vi "Write Pages Properties.vi"(8 "Error In":errorcluster, 10 "All Pages Properties":T10(array[cluster]), 11 "Custom Device .NET Ref In":refnum<k24>) -> (0 "Error Out":errorcluster, 3 "Custom Device .NET Ref Out":refnum<k24>)   [LabVIEW 2015, in "VeriStand Custom Device XML Parser.lvlib"]
doc: "Write the properties for all items of a page then writes the array of pages to the custom device"
uses:
  VeriStand Custom Device XML Parser.lvlib
  NationalInstruments.VeriStand.XMLReader
  XML Controls/Page Properties.ctl
  XML Controls/Path Cluster.ctl
  XML Controls/Help File Properties.ctl
  XML Controls/ActionVIs Properties.ctl
  XML Controls/ButtonLists Properties.ctl
  XML Controls/Button Type.ctl
  XML Controls/Dependency Properties.ctl
  XML Controls/RunTimeMenus Properties.ctl
  XML Controls/Execution Types.ctl
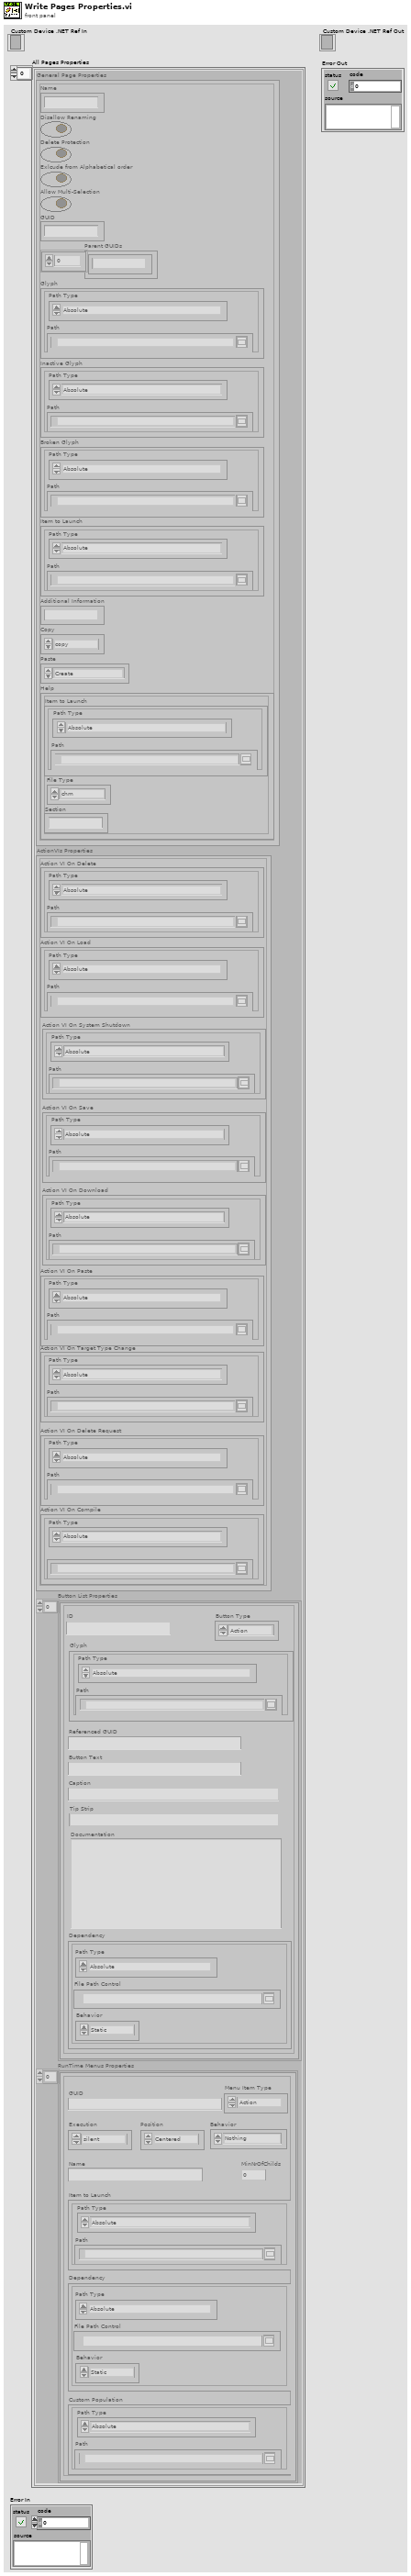
[diagram p1: front panel]
types:
  T1 = typedef "VeriStand Custom Device XML Parser.lvlib/Page Properties.ctl" = cluster{"Name":string, "Disallow Renaming":bool, "Delete Protection":bool, "Exlcude from Alphabetical order":bool, "Allow Multi-Selection":bool, "GUID":string, "Parent GUIDs":string[], "Glyph":T2, "Inactive Glyph":T2, "Broken Glyph":T2, "Item to Launch":T2, "Additional Information":string, "Copy":enum16{"copy", "disabled"}, "Paste":enum16{"Create", "CreatIfNotExists_GUID", "CreatIfNotExists_Name", "Replace", "Dialog"}, "Help":T3}
  T2 = typedef "VeriStand Custom Device XML Parser.lvlib/Path Cluster.ctl" = cluster{"Path":path, "Path Type":enum16{"Absolute", "To Base", "To Common Doc Dir", "To Application Data Dir"}}
  T3 = typedef "VeriStand Custom Device XML Parser.lvlib/Help File Properties.ctl" = cluster{"Item to Launch":T2, "Section":string, "File Type":enum16{"chm", "other"}}
  T4 = typedef "VeriStand Custom Device XML Parser.lvlib/ActionVIs Properties.ctl" = cluster{"Action VI On Delete":T2, "Action VI On Load":T2, "Action VI On Paste":T2, "Action VI On Target Type Change":T2, "Action VI On Delete Request":T2, "Action VI On Compile":T2, "Action VI On System Shutdown":T2, "Action VI On Save":T2, "Action VI On Download":T2}
  T5 = typedef "VeriStand Custom Device XML Parser.lvlib/ButtonLists Properties.ctl" = cluster{"ID":string, "Glyph":T2, "Button Type":T6, "Referenced GUID":string, "Button Text":string, "Caption":string, "Tip Strip":string, "Documentation":string, "Dependency":T7}
  T6 = typedef "VeriStand Custom Device XML Parser.lvlib/Button Type.ctl" = enum16{"Action", "Dialog", "Page", "Notification", "Separator"}
  T7 = typedef "VeriStand Custom Device XML Parser.lvlib/Dependency Properties.ctl" = cluster{"File Path Control":path, "Path Type":enum16{"Absolute", "To Base", "To Common Doc Dir", "To Application Data Dir"}, "Behavior":enum16{"Static", "Dynamic"}}
  T8 = typedef "VeriStand Custom Device XML Parser.lvlib/RunTimeMenus Properties.ctl" = cluster{"GUID":string, "Execution":T9, "MinNrOfChilds":u32, "Name":string, "Item to Launch":T2, "Dependency":T7, "Custom Population":T2, "Menu Item Type":enum16{"Action", "VI", "Separator", "Custom"}, "Behavior":enum16{"Nothing", "Open Front Panel"}, "Position":enum16{"Centered", "Mouse Pointer"}}
  T9 = typedef "VeriStand Custom Device XML Parser.lvlib/Execution Types.ctl" = enum16{"silent", "modal", "floating", "default"}
  T10 = cluster{"General Page Properties":T1, "ActionVIs Properties":T4, "Button List Properties":T5[], "RunTime Menus Properties":T8[]}[]
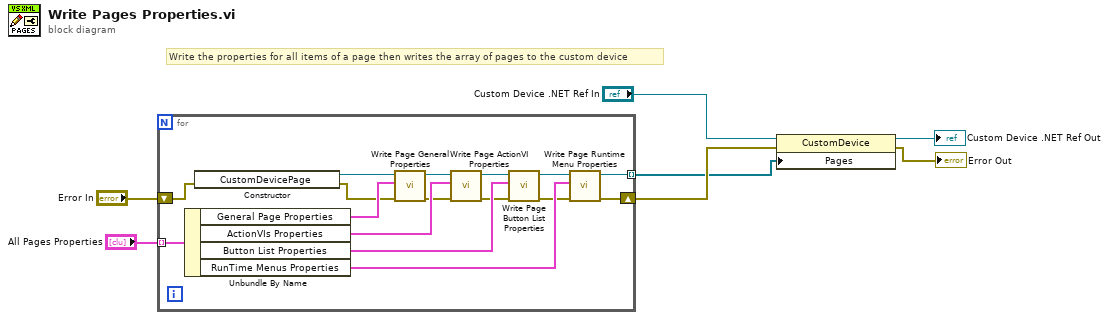
[diagram p0: block diagram]
diagram:
  # "Write the properties for all items of a page then writes the array of pages to the custom device"
  n1 = for {
    tunnel: "All Pages Properties" -> [w23] mode=indexing
    shift-right: [w8] -> w7
    shift-left: "Error In" -> [w20]
    tunnel: [w9] -> w6 mode=indexing
    n2 = Unbundle By Name(w23) -> ("General Page Properties"=w22:T1, "ActionVIs Properties"=w17:T4, "Button List Properties"=w15:T5[], "RunTime Menus Properties"=w12:T8[])
    n3 = constructor class="CustomDevicePage"(error in=w20) -> (reference out=w21:refnum<k24>, error out=w19:errorcluster)  [unwired: 2 in, 1 out]
    n4 = call "Write Page General Properties.vi"("Error In"=w19, "General Page Properties"=w22, "Custom Device Page .NET Ref In"=w21) -> ("Error Out"=w16:errorcluster, "Custom Device Page .NET Ref Out"=w18:refnum<k24>)  [unwired: 7 in]
    n5 = call "Write Page ActionVI Properties.vi"("Error In"=w16, "ActionVIs Properties"=w17, "Custom Device Page .NET Ref In"=w18) -> ("Error Out"=w14:errorcluster, "Custom Device Page .NET Ref Out"=w13:refnum<k24>)  [unwired: 7 in]
    n6 = call "Write Page Button List Properties.vi"("Error In"=w14, "Button List Properties"=w15, "Custom Device Page .NET Ref In"=w13) -> ("Error Out"=w11:errorcluster, "Custom Device Page .NET Ref Out"=w10:refnum<k24>)  [unwired: 7 in]
    n7 = call "Write Page Runtime Menu Properties.vi"("Error In"=w11, "RunTime Menus Properties"=w12, "Custom Device Page .NET Ref In"=w10) -> ("Error Out"=w8:errorcluster, "Custom Device Page .NET Ref Out"=w9:refnum<k24>)  [unwired: 7 in]
  }
  n8 = property class="CustomDevice"(reference="Custom Device .NET Ref In", error in=w7, "Pages"=w6) -> (reference out=→"Custom Device .NET Ref Out":refnum<k24>, error out=→"Error Out":errorcluster)
